vi "AMI.vi"(0 "VISA resource name":refnum<visa-resource-name>, 11 "error in":errorcluster) -> (4 "VISA resource name out":refnum<visa-resource-name>, 6 "Information":string, 8 "Model Name":string, 10 "Version-Revision":string, 14 "Responce (original)":string, 15 "error out":errorcluster)   [LabVIEW 2016, in "Samwontech TEMP2xxx.lvlib"]
doc: "AMI Command is used to get the controller own information"
uses:
  <instrlib>/Samwontech TEMP2xxx/Samwontech TEMP2xxx.lvlib
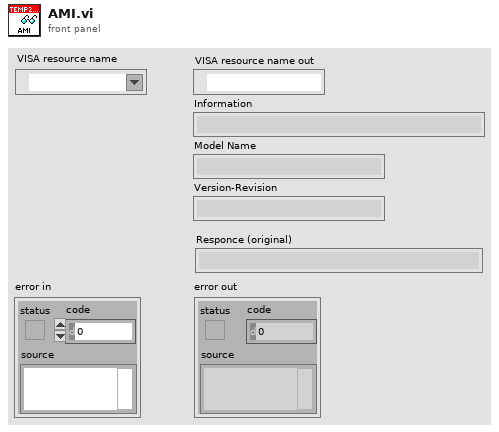
[diagram p1: front panel]
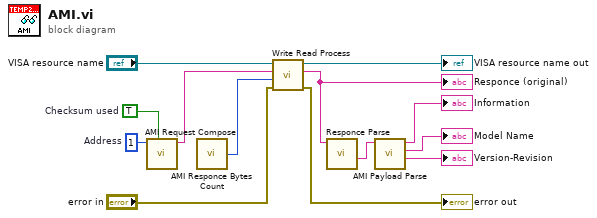
[diagram p0: block diagram]
diagram:
  w12 = TRUE  # Checksum used
  w13 = u8 1  # Address
  n1 = call <instrlib>:"AMI Request Compose.vi"("Checksum used"=w12, "Address"=w13) -> ("Request"=w10:string)  [unwired: 8 in, 1 out]
  n2 = call <instrlib>:"AMI Responce Bytes Count.vi"() -> ("Bytes Count"=w7:u32)
  n3 = call <instrlib>:"Write Read Process.vi"("error in (no error)"="error in", "Responce Bytes Count Required"=w7, "Request"=w10, "VISA Refnum in"="VISA resource name") -> ("error out"=→"error out":errorcluster, "Responce"=w6:string, "VISA Refnum out"=→"VISA resource name out":refnum<visa-resource-name>)  [unwired: 5 in]
  "Responce (original)" <- w6
  n4 = call <instrlib>:"Responce Parse.vi"("Responce"=w6) -> ("Payload"=w5:string)  [unwired: 6 in, 4 out]
  n5 = call <instrlib>:"AMI Payload Parse.vi"("Payload"=w5) -> ("Version-Revision"=→"Version-Revision":string, "Model Name"=→"Model Name":string, "Information"=→"Information":string)  [unwired: 8 in]
